vi "Get Template.vi"(8 "error in (no error)":errorcluster, 10 "id":u32, 11 "eLab in":refnum<class "PL eLabFTW Client.lvclass">) -> (0 "error out":errorcluster, 2 "template":T1 {"lock"."datetime" format="%<%X\n%x>T"}, 3 "eLab out":refnum<class "PL eLabFTW Client.lvclass">)   [LabVIEW 2015, in "PL eLabFTW Client.lvclass"]
doc: "Gets template with the specified id."
uses:
  PL eLabFTW Client.lvclass
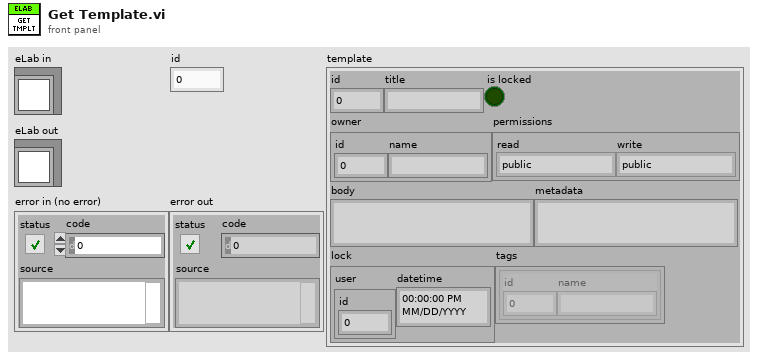
[diagram p1: front panel]
types:
  T1 = cluster{"id":u32, "title":string, "is locked":bool, "owner":cluster{"id":u32, "name":string}, "permissions":cluster{"read":enum16{"public", "organization", "team", "owner and admins", "owner"}, "write":enum16{"public", "organization", "team", "owner and admins", "owner"}}, "body":string, "metadata":string, "lock":cluster{"user":cluster{"id":u32}, "datetime":timestamp}, "tags":cluster{"id":u32, "name":string}[]}
  T2 = cluster{"id":string, "title":string, "body":string, "userid":string, "canread":string, "canwrite":string, "locked":string, "lockedby":string, "lockedwhen":string, "fullname":string, "metadata":string, "state":string, "tags":string, "tags_id":string}
  T3 = cluster{"id":i32, "title":i32, "body":i32, "userid":i32, "canread":i32, "canwrite":i32, "locked":i32, "lockedby":i32, "lockedwhen":i32, "fullname":i32, "metadata":i32, "state":i32, "tags":i32, "tags_id":i32}
  T4 = cluster{"id":bool, "title":bool, "body":bool, "userid":bool, "canread":bool, "canwrite":bool, "locked":bool, "lockedby":bool, "lockedwhen":bool, "fullname":bool, "metadata":bool, "state":bool, "tags":bool, "tags_id":bool}
  T5 = enum16{"public", "organization", "team", "owner and admins", "owner"}
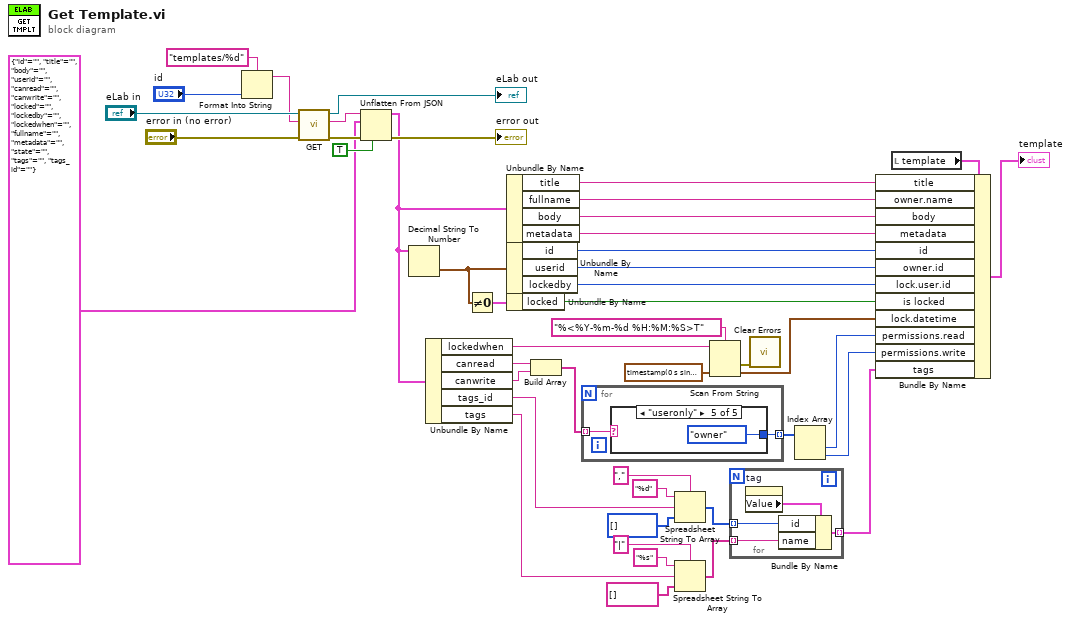
[diagram p0: block diagram]
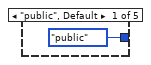
[diagram p2: hidden frame]
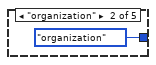
[diagram p3: hidden frame]
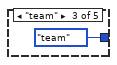
[diagram p4: hidden frame]
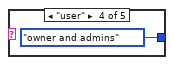
[diagram p5: hidden frame]
diagram:
  n1 = Format Into String(format string="templates/%d", "id") -> (resulting string=w39:string)  [unwired: 2 in, 1 out]
  n2 = call "GET.vi"("error in (no error)"="error in (no error)", "relative URL"=w39, "eLab in"="eLab in") -> ("error out"=w43:errorcluster, "response body"=w8:string, "eLab out"=→"eLab out":refnum<class "PL eLabFTW Client.lvclass">)  [unwired: 6 in]
  n3 = Unflatten From JSON(JSON string=w8, type and defaults=T2 {"id"="", "title"="", "body"="", "userid"="", "canread"="", "canwrite"="", "locked"="", "lockedby"="", "lockedwhen"="", "fullname"="", "metadata"="", "state"="", "tags"="", "tags_id"=""}, default null elements? (F)=TRUE, error in (no error)=w43) -> (value=w19:T2, error out=→"error out":errorcluster)  [unwired: 3 in]
  n4 = Decimal String To Number(string=w19) -> (number=w32:T3)  [unwired: 2 in, 1 out]
  n5 = Unbundle By Name(w19) -> ("lockedwhen"=w5:string, "canread"=w29:string, "canwrite"=w28:string, "tags_id"=w12:string, "tags"=w11:string)
  n6 = Not Equal To 0?(x=w32) -> (x != 0?=w31:T4)
  n7 = Unbundle By Name(w19) -> ("title"=w36:string, "fullname"=w35:string, "body"=w24:string, "metadata"=w23:string)
  n8 = Unbundle By Name(w32) -> ("id"=w34:i32, "userid"=w33:i32, "lockedby"=w22:i32)
  n9 = Unbundle By Name(w31) -> ("locked"=w30:bool)
  n10 = Build Array(w29, w28) -> (w27:string[])
  n11 = for {
    tunnel: w27 -> [w48] mode=indexing
    tunnel: [w47] -> w26 mode=indexing
    n12 = case shown="\"useronly\"" w48 {
      tunnel: [T5."public" ("permissions.read") T5."organization" ("permissions.read") T5."team" ("permissions.read") T5."owner and admins" ("permissions.read") T5."owner" ("permissions.read")] -> w47
      frame "public", Default {
      }
      frame "organization" {
      }
      frame "team" {
      }
      frame "user" {
      }
      frame "useronly" {
      }
    }
  }
  n13 = Spreadsheet String To Array(delimiter (Tab)=",", format string="%d", spreadsheet string=w12, array type (2D Dbl)=u32[] []) -> (array=w10:u32[])
  n14 = Spreadsheet String To Array(delimiter (Tab)="|", format string="%s", spreadsheet string=w11, array type (2D Dbl)=string[] []) -> (array=w9:string[])
  n15 = Scan From String(format string="%<%Y-%m-%d %H:%M:%S>T", input string=w5, default 1=timestamp(0 s since 1904-01-01) ("from")) -> (error out=w7:errorcluster, output 1=w4:timestamp)  [unwired: 2 in, 2 out]
  n16 = for {
    tunnel: [w56] -> w1 mode=indexing
    tunnel: w10 -> [w55] mode=indexing
    tunnel: w9 -> [w54] mode=indexing
    n17 = property on="tag" class="Clust (strict)"() -> ("Value"=w57:cluster{"id":u32, "name":string})  [unwired: 2 in, 2 out]
    n18 = Bundle By Name(cluster=w57, "id"=w55, "name"=w54) -> (w56:cluster{"id":u32, "name":string})
  }
  n19 = call <vilib>:"Clear Errors.vi"("error in (no error)"=w7) -> ()  [unwired: 5 in, 2 out]
  n20 = Index Array(array=w26) -> (element #1=w3:T5, element #2=w2:T5)  [unwired: 2 in]
  n21 = local read "template"() -> (w21:T1)
  n22 = Bundle By Name(cluster=w21, "title"=w36, "owner.name"=w35, "body"=w24, "metadata"=w23, "id"=w34, "owner.id"=w33, "lock.user.id"=w22, "is locked"=w30, "lock.datetime"=w4, "permissions.read"=w3, "permissions.write"=w2, "tags"=w1) -> (→"template":T1)
